vi "Position Control Panel Button.vi"(8 "error in (no error)":errorcluster, 11 "Button Ref":refnum<vi>) -> (0 "error out":errorcluster)   [LabVIEW 2014]
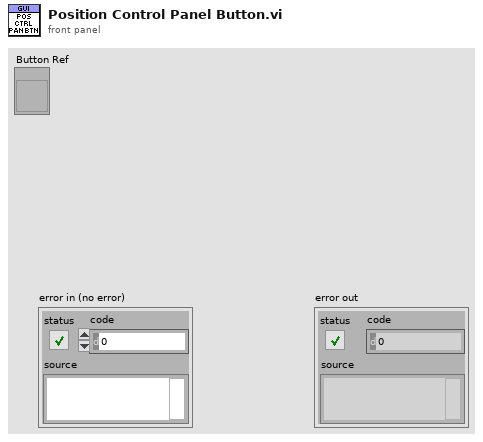
[diagram p1: front panel]
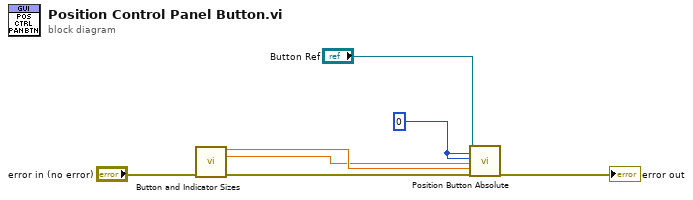
[diagram p0: block diagram]
diagram:
  w5 = 0 ("Left Offset (px)")
  n1 = call "Button and Indicator Sizes.vi"("error in (no error)"="error in (no error)") -> ("Button Width"=w2:dbl, "Button Height"=w1:dbl, "error out"=w3:errorcluster)  [unwired: 10 in, 2 out]
  n2 = call "Position Button Absolute.vi"("Button Ref"="Button Ref", "Left Offset (px)"=w5, "Top Offste (px)"=w5, "Height (px)"=w1, "Width (px)"=w2, "Error In"=w3) -> ("Error Out"=→"error out":errorcluster)  [unwired: 13 in]
